vi "Get Next.vi"(0 "Loop in":refnum<class "Loop.lvclass">, 1 "Linked List Ref":refnum<data-value>, 5 "Active Unique ID":string, 9 "Active Element Index":i32, 11 "error in (no error)":errorcluster) -> (3 "Linked List Ref out":refnum<data-value>, 4 "Executioner out":refnum<class "Executioner.lvclass">, 6 "Active Unique ID out":string, 8 "Test Executive Ref out":refnum<data-value>, 10 "Active Element Index out":i32, 12 "Found":bool, 13 "Complete":bool, 14 "Stop":bool, 15 "error out":errorcluster)   [LabVIEW 2019, in "Test Executive.lvlib" / "Loop.lvclass"]
uses:
  <vilib>/gpm_packages/@cs/test-executive/Source/Test Executive/Loop/Loop.lvclass
  C:/Program Files/National Instruments/LabVIEW 2019/vi.lib/gpm_packages/@cs/test-executive/Source/Test Executive/Executioner/Executioner.lvclass
  <vilib>/gpm_packages/@cs/test-executive/Source/Test Executive/Executioner/Executioner.lvclass
  <vilib>/gpm_packages/@cs/linked-list/Source/Linked List/ILinkedList/ILinked List.lvclass
  <vilib>/gpm_packages/@cs/test-executive/Source/Test Executive/ITestExecutive/ITest Executive.lvclass
  861e28d1-00f5-42f5-88ec-2f811e324c0a.vi
  92e84ae4-1d7a-4e08-891f-f0103df7ce27.vi
  2833b21d-d3e9-4ddc-b049-63a319df379c.vi
  98228b8a-282e-49cd-8fcb-6487c253d078.vi
  478ee926-a488-4361-bcbb-bc1b8ad98273.vi
  e9f0fb3d-5f16-465a-b432-d1c3f7e1e47d.vi
  <vilib>/gpm_packages/@cs/linked-list/Source/Linked List/Linked List Ref/Linked List Ref.lvclass
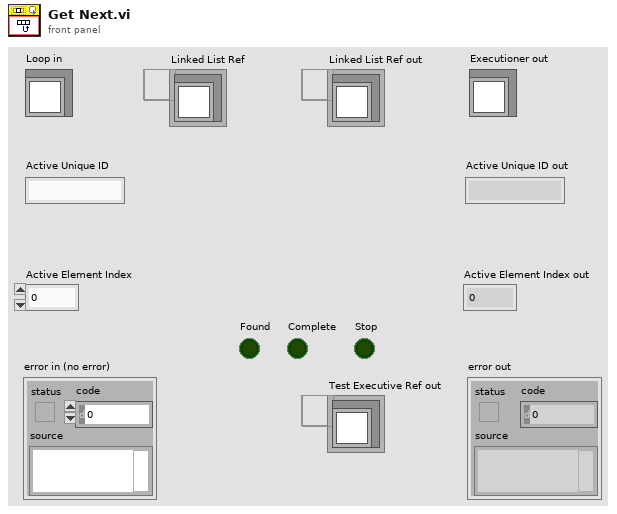
[diagram p1: front panel]
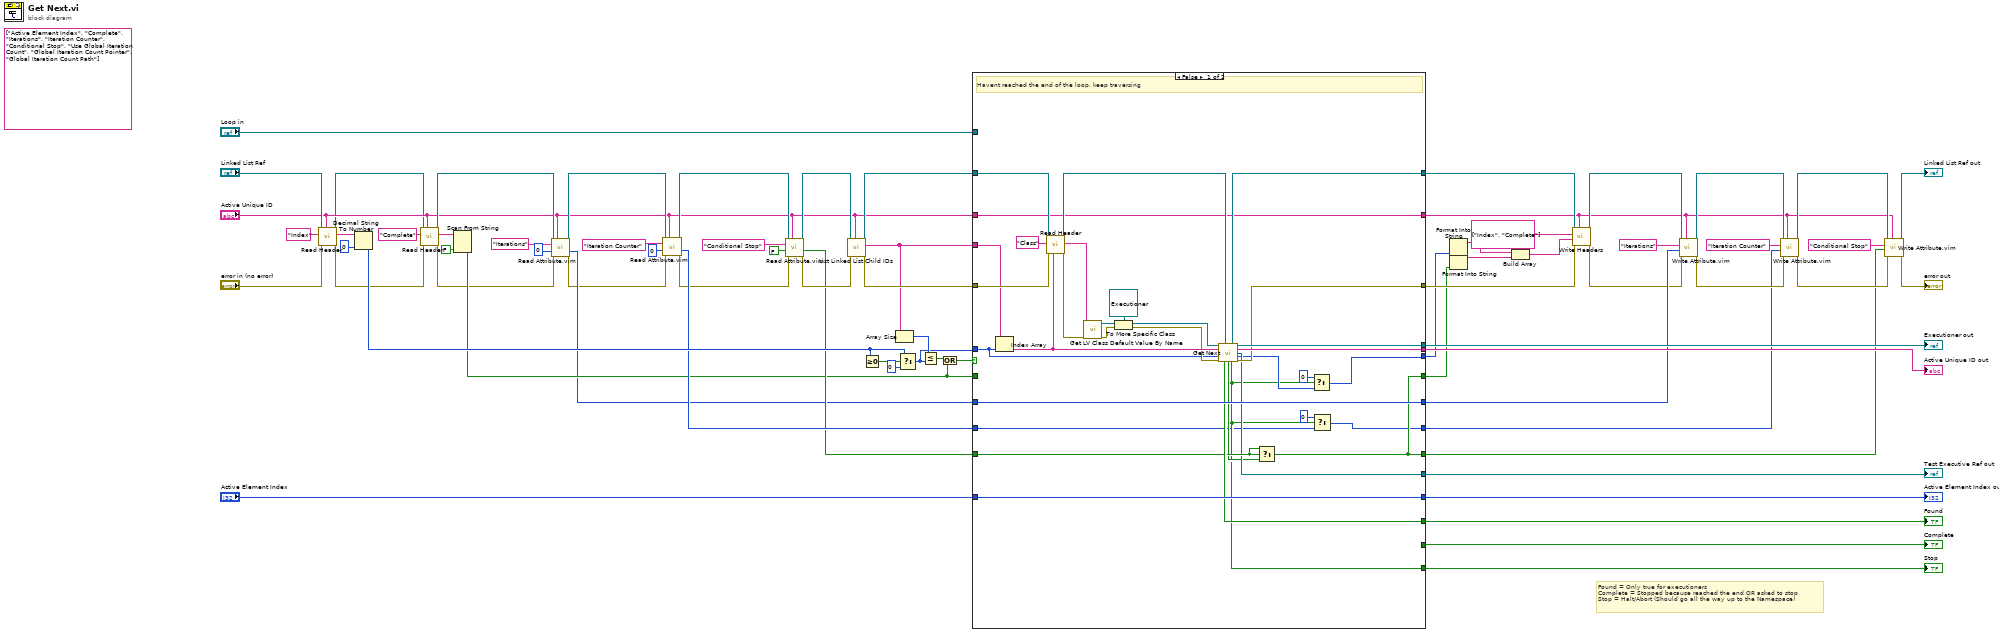
[diagram p0: block diagram]
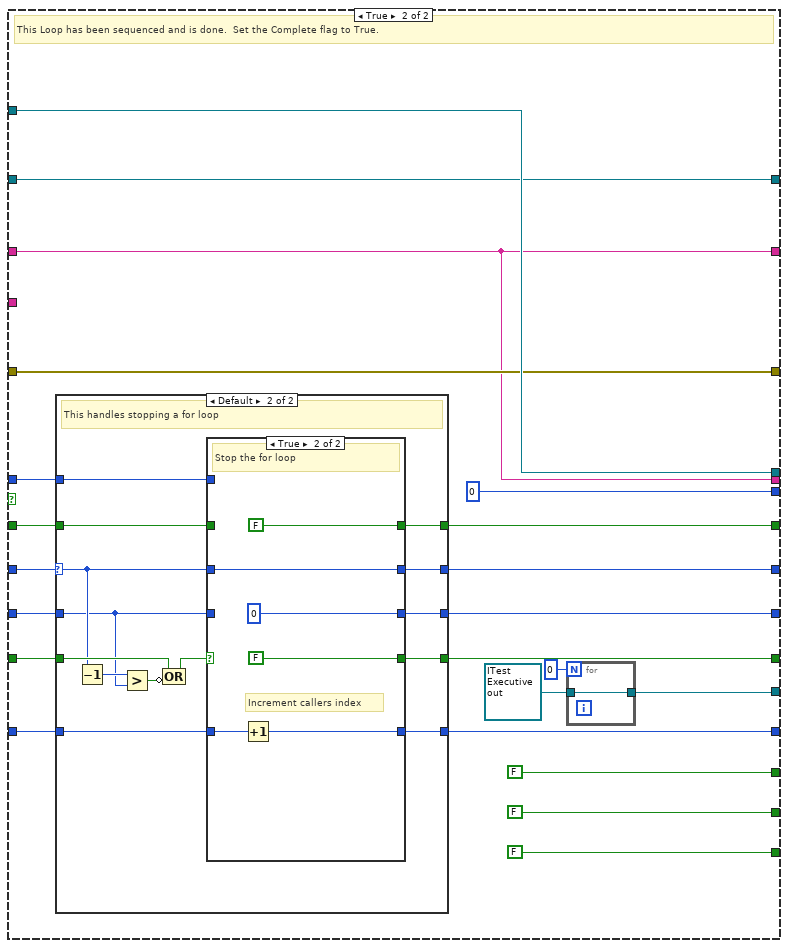
[diagram p2: hidden frame]
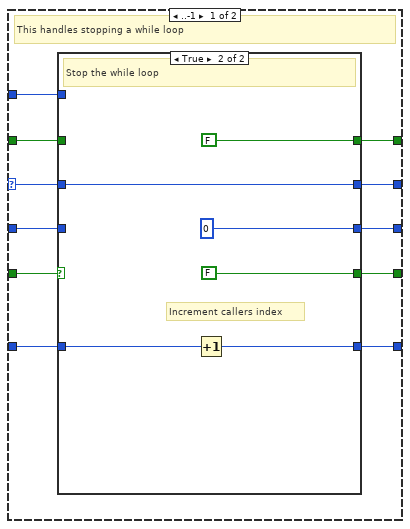
[diagram p3: hidden frame]
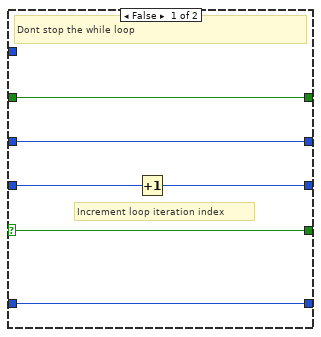
[diagram p4: hidden frame]
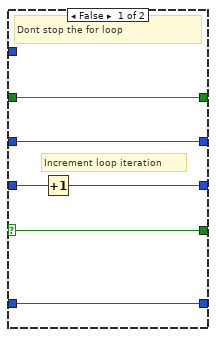
[diagram p5: hidden frame]
diagram:
  (unwired) string[] ["Active Element Index", "Complete", "Iterations", "Iteration Counter", "Conditional Stop", "Use Global Iteration Count", "Global Iteration Count Pointer", "Global Iteration Count Path"] ("Attribute Names")
  # "Found = Only true for executioners\nComplete = Stopped because reached the end OR asked to stop\nStop = Halt/Abort (Should go all the way up to the Namespace)"
  n1 = call <vilib>:"Read Header.vi"("Linked List ID"="Active Unique ID", "error in (no error)"="error in (no error)", "Header Name"="Index" ("Attribute Name"), "Linked List Ref"="Linked List Ref") -> ("error out"=w6:errorcluster, "Header Value"=w12:string, "Linked List Ref out"=w7:refnum<data-value>)  [unwired: 4 in, 1 out]
  n2 = Decimal String To Number(string=w12, default (0L)=0 ("Attribute")) -> (number=w59:i32)  [unwired: 1 in, 1 out]
  n3 = call <vilib>:"Read Header.vi"("Linked List ID"="Active Unique ID", "error in (no error)"=w6, "Header Name"="Complete" ("Attribute Name"), "Linked List Ref"=w7) -> ("error out"=w18:errorcluster, "Header Value"=w9:string, "Linked List Ref out"=w22:refnum<data-value>)  [unwired: 4 in, 1 out]
  n4 = Scan From String(input string=w9, default 1=FALSE) -> (output 1=w44:bool)  [unwired: 3 in, 3 out]
  n5 = call "Read Attribute.vim"("Linked List Ref"=w22, "Linked List ID"="Active Unique ID", "Attribute Name"="Iterations", "Type"=0, "error in (no error)"=w18) -> ("Linked List Ref out"=w21:refnum<data-value>, "Attribute"=w17:i32, "error out"=w16:errorcluster)  [unwired: 5 in, 3 out]
  n6 = call "Read Attribute.vim"("Linked List Ref"=w21, "Linked List ID"="Active Unique ID", "Attribute Name"="Iteration Counter", "Type"=0, "error in (no error)"=w16) -> ("Linked List Ref out"=w34:refnum<data-value>, "Attribute"=w55:i32, "error out"=w33:errorcluster)  [unwired: 5 in, 3 out]
  n7 = call "Read Attribute.vim"("Linked List Ref"=w34, "Linked List ID"="Active Unique ID", "Attribute Name"="Conditional Stop", "Type"=FALSE, "error in (no error)"=w33) -> ("Linked List Ref out"=w65:refnum<data-value>, "Attribute"=w54:bool, "error out"=w64:errorcluster)  [unwired: 5 in, 3 out]
  n8 = call <vilib>:"List Linked List Child IDs.vi"("Linked List ID"="Active Unique ID", "error in (no error)"=w64, "Linked List Ref"=w65) -> ("error out"=w57:errorcluster, "Child IDs"=w53:string[], "Linked List Ref out"=w58:refnum<data-value>)  [unwired: 6 in]
  n9 = Greater Or Equal To 0?(x=w59) -> (x >= 0?=w63:bool)
  n10 = Array Size(array=w53) -> (size(s)=w60:i32)
  n11 = Select(t=w59, s=w63, f=0) -> (s? t:f=w52:i32)
  n12 = Less Or Equal?(x=w60, y=w52) -> (x <= y?=w61:bool)
  n13 = Or(x=w61, y=w44) -> (x .or. y?=w56:bool)
  n14 = case shown="False" w56 {
    tunnel: w58 -> [w96 w124]
    tunnel: [w93 w124] -> w42
    tunnel: [w82 w125] -> w41
    tunnel: w57 -> [w95 w125]
    tunnel: w17 -> [w90 w120]
    tunnel: w55 -> [w73 w118]
    tunnel: w54 -> [w85 w119]
    tunnel: w53 -> [w92 _]
    tunnel: w52 -> [w91 w122]
    tunnel: [w90 w112] -> w37
    tunnel: [w72 w111] -> w29
    tunnel: [w76 0 ("Active Element Index out")] -> w40
    tunnel: [w89 w109] -> w45
    tunnel: [w88 w126] -> w46
    tunnel: "Loop in" -> [_ w126]
    tunnel: "Active Element Index" -> [w87 w117]
    tunnel: [w87 w114] -> w49
    tunnel: [_ FALSE] -> w48
    tunnel: [w74 FALSE] -> w47
    tunnel: "Active Unique ID" -> [w84 w109]
    tunnel: w44 -> [_ w121]
    tunnel: [w86 FALSE] -> w43
    tunnel: [w81 w113] -> w39
    tunnel: [w81 w110] -> w23
    tunnel: [w84 w109] -> w14
    tunnel: [w80 w106] -> w1
    frame False {
      # "Havent reached the end of the loop, keep traversing"
      n15 = Index Array(array=w92, index=w91) -> (element=w103:string)
      n16 = call <vilib>:"Read Header.vi"("Linked List ID"=w103, "error in (no error)"=w95, "Header Name"="Class", "Linked List Ref"=w96) -> ("error out"=w83:errorcluster, "Header Value"=w102:string, "Linked List Ref out"=w94:refnum<data-value>)  [unwired: 4 in, 1 out]
      n17 = call <vilib>:"Get LV Class Default Value By Name.vi"("error in (no error)"=w83, "class name"=w102) -> ("error out"=w98:errorcluster, "object"=w101:refnum<class>)  [unwired: 8 in]
      n18 = To More Specific Class(target class=refnum<class "Executioner.lvclass"> refnum ("Test Executive.lvlib:Executioner.lvclass"), reference=w101, error in=w98) -> (specific class reference=w97:refnum<class "Executioner.lvclass">, error out=w99:errorcluster)
      n19 = call-dynamic "Get Next.vi"("Executioner in"=w97, "Linked List Ref"=w94, "Active Unique ID"=w103, "Active Element Index"=w91, "error in (no error)"=w99) -> ("Linked List Ref out"=w93:refnum<data-value>, "Executioner out"=w88:refnum<class "Executioner.lvclass">, "Active Unique ID out"=w89:string, "Test Executive Ref out"=w80:refnum<data-value>, "Active Element Index out"=w77:i32, "Found"=w86:bool, "Complete"=w79:bool, "Stop"=w74:bool, "error out"=w82:errorcluster)  [unwired: 2 in]
      n20 = Select(t=w85, s=w85, f=w79) -> (s? t:f=w81:bool)
      n21 = Select(t=0, s=w74, f=w77) -> (s? t:f=w76:i32)
      n22 = Select(t=0, s=w74, f=w73) -> (s? t:f=w72:i32)
    }
    frame True {
      # "This Loop has been sequenced and is done.  Set the Complete flag to True."
      n23 = case shown="Default" w120 {
        selector: w120 -> [w134 w152]
        tunnel: w119 -> [w138 w154]
        tunnel: w118 -> [w133 w151]
        tunnel: [w137 w164] -> w114
        tunnel: w117 -> [w136 w163]
        tunnel: w122 -> [w130 w159]
        tunnel: [w135 w162] -> w112
        tunnel: [w132 w161] -> w110
        tunnel: [w131 w160] -> w111
        tunnel: [w129 w158] -> w113
        tunnel: w121 -> [w128 w157]
        frame ..-1 {
          # "This handles stopping a while loop"
          n24 = case shown="True" w138 {
            selector: w138 -> [w140 _]
            tunnel: [w144 w149] -> w137
            tunnel: w136 -> [w144 w150]
            tunnel: [w141 w148] -> w135
            tunnel: w134 -> [w141 w148]
            tunnel: w133 -> [w143 _]
            tunnel: [w140 FALSE] -> w132
            tunnel: [w142 0 ("Numeric")] -> w131
            tunnel: w130 -> [_ _]
            tunnel: [w139 FALSE] -> w129
            tunnel: w128 -> [w139 _]
            frame False {
              # "Increment loop iteration index"
              # "Dont stop the while loop"
              n25 = Increment(x=w143) -> (x+1=w142:i32)
            }
            frame True {
              # "Increment callers index"
              # "Stop the while loop"
              n26 = Increment(x=w150) -> (x+1=w149:i32)
            }
          }
        }
        frame Default {
          # "This handles stopping a for loop"
          n27 = Decrement(x=w152) -> (x-1=w156:i32)
          n28 = Greater?(x=w156, y=w151) -> (0:w155:bool)
          n29 = Compound Arithmetic op=OR(w154, invert w155) -> (w153:bool)
          n30 = case shown="True" w153 {
            selector: w153 -> [w166 _]
            tunnel: [w170 w175] -> w164
            tunnel: w163 -> [w170 w176]
            tunnel: [w167 w174] -> w162
            tunnel: w152 -> [w167 w174]
            tunnel: w151 -> [w169 _]
            tunnel: [w166 FALSE] -> w161
            tunnel: [w168 0 ("Numeric")] -> w160
            tunnel: w159 -> [_ _]
            tunnel: [w165 FALSE] -> w158
            tunnel: w157 -> [w165 _]
            frame False {
              # "Increment loop iteration"
              # "Dont stop the for loop"
              n31 = Increment(x=w169) -> (x+1=w168:i32)
            }
            frame True {
              # "Increment callers index"
              # "Stop the for loop"
              n32 = Increment(x=w176) -> (x+1=w175:i32)
            }
          }
        }
      }
      n33 = for {
        N: 0 -> [_]
        tunnel: refnum<data-value> refnum ("Test Executive Ref out") -> [w127]
        tunnel: [w127] -> w106
      }
    }
  }
  "Executioner out" <- w46
  "Active Unique ID out" <- w45
  "Active Element Index out" <- w49
  "Found" <- w43
  "Complete" <- w48
  "Stop" <- w47
  "Test Executive Ref out" <- w1
  n34 = Format Into String(w40) -> (resulting string=w4:string)  [unwired: 3 in, 1 out]
  n35 = Format Into String(w39) -> (resulting string=w3:string)  [unwired: 3 in, 1 out]
  n36 = Build Array(w4, w3) -> (w2:string[])
  n37 = call <vilib>:"Write Headers.vi"("Linked List ID"=w14, "error in (no error)"=w41, "Header Values"=w2, "Header Names"=string[] ["Index", "Complete"], "Linked List Ref"=w42) -> ("error out"=w36:errorcluster, "Linked List Ref out"=w35:refnum<data-value>)  [unwired: 5 in]
  n38 = call "Write Attribute.vim"("Linked List ID"=w14, "error in (no error)"=w36, "Attribute"=w37, "Attribute Name"="Iterations", "Linked List Ref"=w35) -> ("error out"=w31:errorcluster, "Linked List Ref out"=w32:refnum<data-value>)  [unwired: 3 in, 2 out]
  n39 = call "Write Attribute.vim"("Linked List ID"=w14, "error in (no error)"=w31, "Attribute"=w29, "Attribute Name"="Iteration Counter", "Linked List Ref"=w32) -> ("error out"=w26:errorcluster, "Linked List Ref out"=w28:refnum<data-value>)  [unwired: 3 in, 2 out]
  n40 = call "Write Attribute.vim"("Linked List ID"=w14, "error in (no error)"=w26, "Attribute"=w23, "Attribute Name"="Conditional Stop", "Linked List Ref"=w28) -> ("error out"=→"error out":errorcluster, "Linked List Ref out"=→"Linked List Ref out":refnum<data-value>)  [unwired: 3 in, 2 out]
